vi "動態創queue.vi"() -> ()   [LabVIEW 2015]
panel:
  in  "Boolean 3":bool
  in  "Boolean 2":bool
  in  "Boolean":bool
  out "# elements in queue 3":i32
  out "# elements in queue 2":i32
  out "# elements in queue":i32
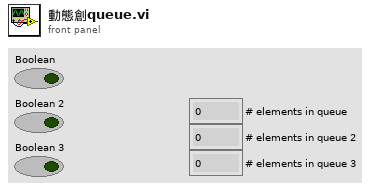
[diagram p1: front panel]
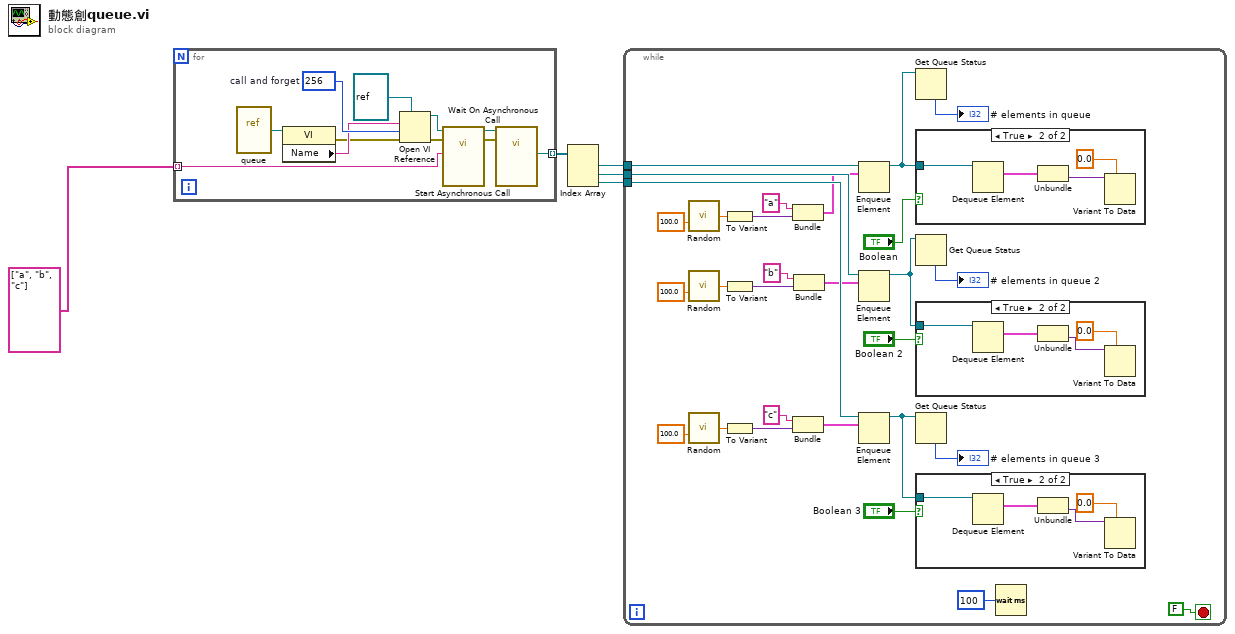
[diagram p0: block diagram]
diagram:
  n1 = for {
    tunnel: string[] ["a", "b", "c"] -> [w10] mode=indexing
    tunnel: [w8] -> w1 mode=indexing
    w16 = 256  # call and forget
    n2 = vi-ref "queue.vi"() -> (w13:refnum<vi>)
    n3 = property class="VI"(reference=w13) -> (error out=w11:errorcluster, "Name"=w12:string)  [unwired: 1 in, 1 out]
    n4 = Open VI Reference(type specifier VI Refnum (for type only)=refnum<vi> refnum, vi path=w12, options=w16, error in (no error)=w11) -> (vi reference=w9:refnum<vi>, error out=w14:errorcluster)  [unwired: 2 in]
    n5 = call-by-ref "Start Asynchronous Call"(reference=w9, error in=w14, "name"=w10) -> (reference out=w7:refnum<vi>, error out=w6:errorcluster)  [unwired: 10 in, 1 out]
    n6 = call-by-ref "Wait On Asynchronous Call"(reference=w7, error in=w6) -> ("queue out"=w8:refnum<queue>)  [unwired: 11 in, 2 out]
  }
  n7 = Index Array(array=w1) -> (element #1=w3:refnum<queue>, element #2=w2:refnum<queue>, element #3=w4:refnum<queue>)  [unwired: 3 in]
  n8 = while {
    tunnel: w4 -> [w45]
    tunnel: w3 -> [w44]
    tunnel: w2 -> [w43]
    stop <- FALSE stop-if-true
    n9 = call <userlib>:"Random.vi"("Max"=100.0) -> ("Random"=w20:dbl)  [unwired: 14 in]
    n10 = call <userlib>:"Random.vi"("Max"=100.0) -> ("Random"=w21:dbl)  [unwired: 14 in]
    n11 = call <userlib>:"Random.vi"("Max"=100.0) -> ("Random"=w22:dbl)  [unwired: 14 in]
    n12 = To Variant(anything=w20) -> (Variant=w41:variant)
    n13 = To Variant(anything=w21) -> (Variant=w39:variant)
    n14 = To Variant(anything=w22) -> (Variant=w37:variant)
    n15 = Bundle("String"="a", "Variant"=w41) -> (w36:cluster{"String":string, "Variant":variant})  [unwired: 1 in]
    n16 = Bundle("c", "Variant"=w37) -> (w34:cluster{string, "Variant":variant})  [unwired: 1 in]
    n17 = Bundle("b", "Variant"=w39) -> (w35:cluster{string, "Variant":variant})  [unwired: 1 in]
    n18 = Enqueue Element(queue=w44, element=w36) -> (queue out=w33:refnum<queue>)  [unwired: 2 in, 2 out]
    n19 = Enqueue Element(queue=w43, element=w35) -> (queue out=w29:refnum<queue>)  [unwired: 2 in, 2 out]
    n20 = Enqueue Element(queue=w45, element=w34) -> (queue out=w28:refnum<queue>)  [unwired: 2 in, 2 out]
    n21 = Get Queue Status(queue=w33) -> (# elements in queue=→"# elements in queue":i32)  [unwired: 2 in, 7 out]
    n22 = case shown="True" "Boolean" {
      tunnel: w33 -> [_ w57]
      frame False {
      }
      frame True {
        n23 = Dequeue Element(queue=w57) -> (element=w56:cluster{string, variant})  [unwired: 2 in, 3 out]
        n24 = Unbundle(w56) -> (w55:variant)  [unwired: 1 out]
        n25 = Variant To Data(type=0.0 ("Max"), Variant=w55) -> ()  [unwired: 1 in, 2 out]
      }
    }
    n26 = Get Queue Status(queue=w29) -> (# elements in queue=→"# elements in queue 2":i32)  [unwired: 2 in, 7 out]
    n27 = case shown="True" "Boolean 2" {
      tunnel: w29 -> [_ w53]
      frame False {
      }
      frame True {
        n28 = Dequeue Element(queue=w53) -> (element=w52:cluster{string, variant})  [unwired: 2 in, 3 out]
        n29 = Unbundle(w52) -> (w51:variant)  [unwired: 1 out]
        n30 = Variant To Data(type=0.0 ("Max"), Variant=w51) -> ()  [unwired: 1 in, 2 out]
      }
    }
    n31 = Get Queue Status(queue=w28) -> (# elements in queue=→"# elements in queue 3":i32)  [unwired: 2 in, 7 out]
    n32 = case shown="True" "Boolean 3" {
      tunnel: w28 -> [_ w49]
      frame False {
      }
      frame True {
        n33 = Dequeue Element(queue=w49) -> (element=w48:cluster{string, variant})  [unwired: 2 in, 3 out]
        n34 = Unbundle(w48) -> (w47:variant)  [unwired: 1 out]
        n35 = Variant To Data(type=0.0 ("Max"), Variant=w47) -> ()  [unwired: 1 in, 2 out]
      }
    }
    n36 = Wait (ms)(milliseconds to wait=u32 100) -> ()  [unwired: 1 out]
  }
